vi "Normalize_Array.vi"(7 "Normalize? (true)":bool=TRUE, 10 "array":dbl[](array[numeric])) -> (2 "normalized array":dbl[](array[numeric]))   [LabVIEW 2018]
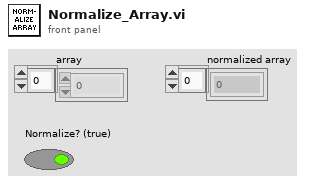
[diagram p1: front panel]
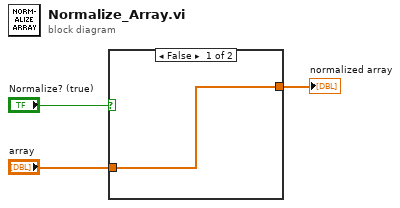
[diagram p0: block diagram]
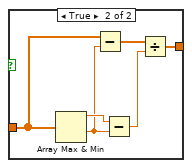
[diagram p2: hidden frame]
diagram:
  n1 = case shown="False" "Normalize? (true)" {
    tunnel: "array" -> [w4 w6]
    tunnel: [w4 w5] -> w2
    frame False {
    }
    frame True {
      n2 = Array Max & Min(array=w6) -> (max value=w10:dbl, min value=w9:dbl)  [unwired: 2 out]
      n3 = Subtract(x=w6, y=w9) -> (x-y=w7:dbl[])
      n4 = Subtract(x=w10, y=w9) -> (x-y=w8:dbl)
      n5 = Divide(x=w7, y=w8) -> (x/y=w5:dbl[])
    }
  }
  "normalized array" <- w2
